vi "Goal Vision Preferences.vi"(9 "Named Controls in":T1, 10 "Operation":enum16{"Save", "Load"}(ring)=enum."Load", 11 "Refnum":T2) -> (2 "Count":i32, 3 "Warnings List":string)   [LabVIEW 2013]
uses:
  <vilib>/Utility/config.llb/Config Data RefNum.ctl
  Named Control.ctl
  <vilib>/Utility/config.llb/NI_LVConfig.lvlib
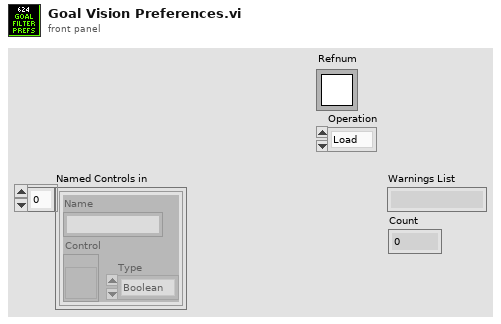
[diagram p1: front panel]
types:
  T1 = typedef "Named Control.ctl" = cluster{"Name":string, "Control":refnum<vi>, "Type":enum16{"Boolean", "Double"}}[]
  T2 = typedef "NI_LVConfig.lvlib/Config Data RefNum.ctl" = refnum<k1>
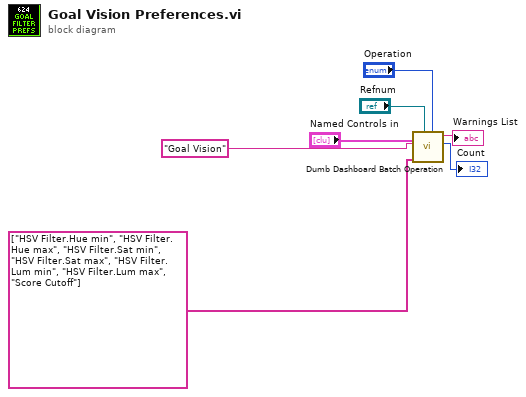
[diagram p0: block diagram]
diagram:
  n1 = call "Dumb Dashboard Batch Operation.vi"("Operation"="Operation", "Refnum in"="Refnum", "Names List"=string[] ["HSV Filter.Hue min", "HSV Filter.Hue max", "HSV Filter.Sat min", "HSV Filter.Sat max", "HSV Filter.Lum min", "HSV Filter.Lum max", "Score Cutoff"], "Section"="Goal Vision", "Named Controls in"="Named Controls in") -> ("Count"=→"Count":i32, "Warnings List"=→"Warnings List":string)  [unwired: 5 in]
